vi "Paramater_analyser_main_file.vi"() -> ()   [LabVIEW 2021]
uses:
  <vilib>/Utility/file.llb/Write Delimited Spreadsheet (DBL).vi
panel:
  out "R-square":dbl format="%#_6e"
  out "Intercept":dbl format="%#_4e"
  out "Resistance (Ohm)":dbl format="%#_4p"
  in  "Estimated Length (mm)":dbl=12.0
  in  "Estimated Width (mm)":dbl=3.0
  out "Double - Voltage":dbl
  out "Double - Current":dbl
  out "First Cycle Reverse Sweep":cluster{"Y":dbl[], "Y":dbl[]}[](graph)
  out "First Cycle Forward Sweep":cluster{"Y":dbl[], "Y":dbl[]}[](graph)
  out "Single - Current":dbl
  out "Single - Voltage":dbl
  out "Recorded_Data":dbl[][][](array[numeric])
  out "WarmUp":dbl[][](array[numeric])
  out "Values Committed":bool
  in  "Press to start":bool
  in  "Set Swe_2_Mode":string(combo)="Single"
  in  "Set Swe_1_Mode":string(combo)="Double"
  in  "SMU1 Terminal":string(combo)="Source"
  in  "Sample Information":string="Synthetic_for_finishing program"
  in  "User":string="Richard"
  out "error out":errorcluster
  in  "VISA resource name":refnum<visa-resource-name>="PA"
  out "DorG_2":string
  out "DorG_1":string
  in  "VIntegration_2":dbl=100.0
  in  "VIntegration_1":dbl=100.0
  out "V_Cst_2 [V]":dbl
  out "V Cst_1 [V]":dbl
  out "V Cst_0 [V]":dbl
  out "V Step_2":dbl
  out "V Step_1":dbl
  out "V Step_0":dbl
  in  "Vvar_2_points":dbl=10.0
  in  "Vvar_1_points":dbl=10.0
  in  "Vvar_0_points":dbl=10.0
  in  "DorG_0":string(combo)="Gate"
  in  "Vvar_2_Stop":dbl=1.0
  in  "Vvar_1_Stop":dbl=1.0
  in  "Vvar_0_Stop":dbl
  in  "Vvar_2_start":dbl
  in  "Vvar_1_start":dbl
  in  "Vvar_0_start":dbl
  in  "# Cycles":dbl=1.0
  in  "Sweep Spacing_2":string(combo)="Linear"
  in  "Sweep Spacing_1":string(combo)="Linear"
  in  "Sweep Spacing_0":string(combo)="Linear"
  in  "VIntegration_0":dbl=100.0
  in  "Gate Current Compliance 2":dbl=1e-06
  in  "Gate Current Compliance 1":dbl=1e-06
  in  "Gate Current Compliance 0":dbl=1e-06
  in  "Drain Current Compliance 2":dbl=0.0001 format="%#_6p"
  in  "Drain Current Compliance 1":dbl=0.01 format="%#_6p"
  in  "Drain Current Compliance":dbl=1e-06
  in  "Sweep 2":bool
  in  "Sweep 0":bool
  in  "Vvar-2_delaytime":dbl
  in  "Vvar_1_delaytime":dbl
  in  "Vvar-0_delaytime":dbl
  in  "Vvar_2_holdtime":dbl
  in  "Vvar_1_holdtime":dbl
  in  "Vvar_0_holdtime":dbl
  out "VISA resource name out":refnum<visa-resource-name>
  in  "error in (no error)":errorcluster
  out "SMU3 Terminal":string
  out "SMU2 Terminal":string
  out "Sweep 2 Point Checker":string
  out "Sweep 2 Pot Check":string
  out "Sweep 1 Point Checker":string
  out "Sweep 1 Pot Check":string
  out "Gate Point number Checker":string
  out "Gate Potential_checker":string
  in  "V_const_2":dbl
  in  "V_const_1":dbl
  in  "V_const_0":dbl
  in  "Vstep2":dbl
  in  "Vstep1":dbl
  in  "Vstep0":dbl
  # "Meta Data"
  # "I(S)"
  # "I(G)"
  # "Voltage"
  # "T(G)"
  # "T(S)"
  # "T(D)"
  # "I(D)"
  # "Warmup is not yet fully implemented"
  # "V Stop"
  # "Sweep Mode"
  # "Delay Time"
  # "Drain/Gate"
  # "V Start"
  # "# Points"
  # "V Step"
  # "V Cst"
  # "Sweep Spacing"
  # "Drain Current Comp"
  # "Gate Current Comp"
  # "Hold Time"
  # "Integration"
  # "Single"
  # "V Stop"
  # "Sweep Mode"
  # "Delay Time"
  # "Drain/Gate"
  # "V Start"
  # "# Points"
  # "V Step"
  # "V Cst"
  # "Sweep Spacing"
  # "Drain Current Comp"
  # "Gate Current Comp"
  # "Hold Time"
  # "Integration"
  # "Operational_placeholders do not modify"
  # "Second_sweep is not yet implemented"
  # "V Stop"
  # "Sweep Mode"
  # "Delay Time"
  # "Drain/Gate"
  # "V Start"
  # "# Points"
  # "V Step"
  # "V Cst"
  # "Sweep Spacing"
  # "Drain Current Comp"
  # "Gate Current Comp"
  # "Hold Time"
  # "Integration"
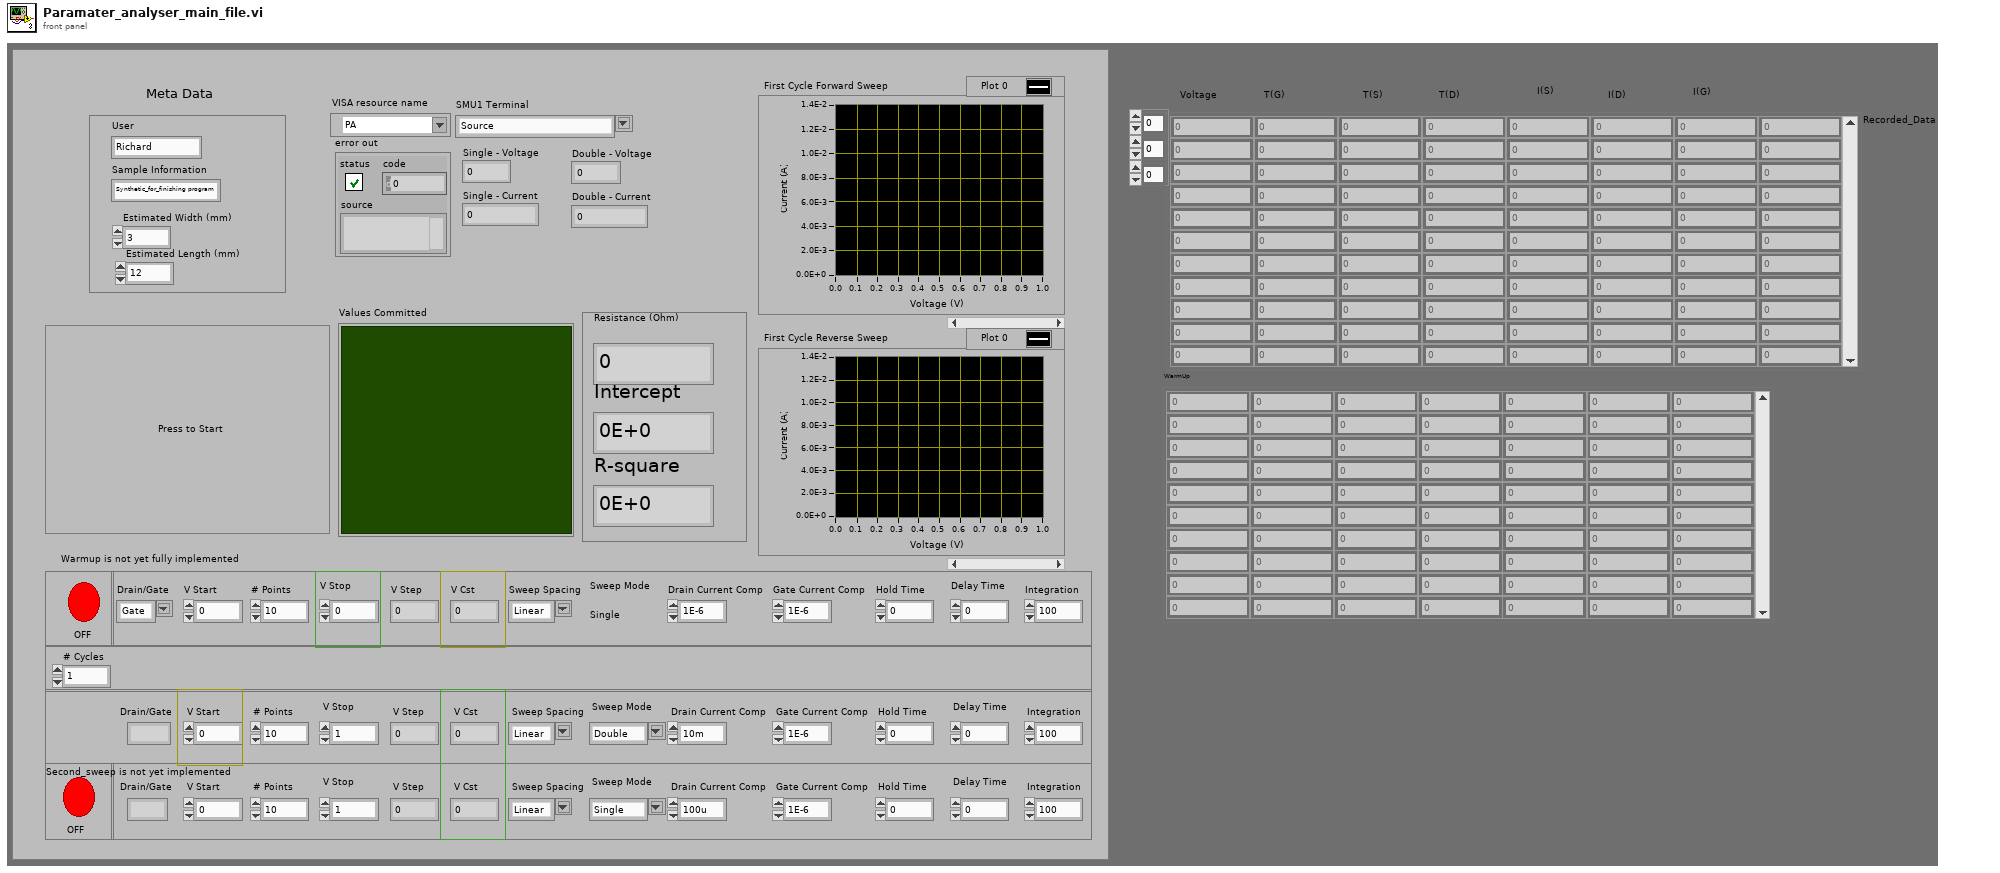
[diagram p1: front panel]
types:
  T1 = enum16{"open", "replace", "create", "open or create", "replace or create", "replace or create with confirmation"}
  T2 = cluster{"DorG_0":string, "Vvar_0_start":dbl, "Vstep0":dbl, "Vvar_0_Stop":dbl, "V_const_0":dbl, "Drain Current Compliance":dbl, "Gate Current Compliance 0":dbl, "Vvar_0_holdtime":dbl, "Vvar-0_delaytime":dbl, "Output Integration":dbl, string, "Sweep Spacing_0":string}
  T3 = cluster{string, "Vvar_1_start ":dbl, "Vstep1":dbl, "Vvar_1_Stop":dbl, "V_const_1":dbl, "Drain Current Compliance 1":dbl, "Gate Current Compliance 1":dbl, "Vvar_1_holdtime":dbl, "Vvar_1_delaytime":dbl, "Output Integration":dbl, "Set Swe_1_Mode":string, "Sweep Spacing_1":string}
  T4 = cluster{string, "Vvar_2_start":dbl, "Vstep2":dbl, "Vvar_2_Stop":dbl, "V_const_2":dbl, "Drain Current Compliance 2":dbl, "Gate Current Compliance 2":dbl, "Vvar_2_holdtime":dbl, "Vvar-2_delaytime":dbl, "Output Integration":dbl, "Set Swe_2_Mode":string, "Sweep Spacing_2":string}
  T5 = cluster{"DorG":string, "Vvar_start":dbl, "Vvar_step":dbl, "Vvar_Stop":dbl, "V_const ":dbl, "Drain Current Compliance":dbl, "Gate Current Compliance":dbl, "Vvar_holdtime":dbl, "Vvar_delaytime":dbl, "IntPts":dbl, "Set Swe_Mode":string, "Sweep Spacing":string}
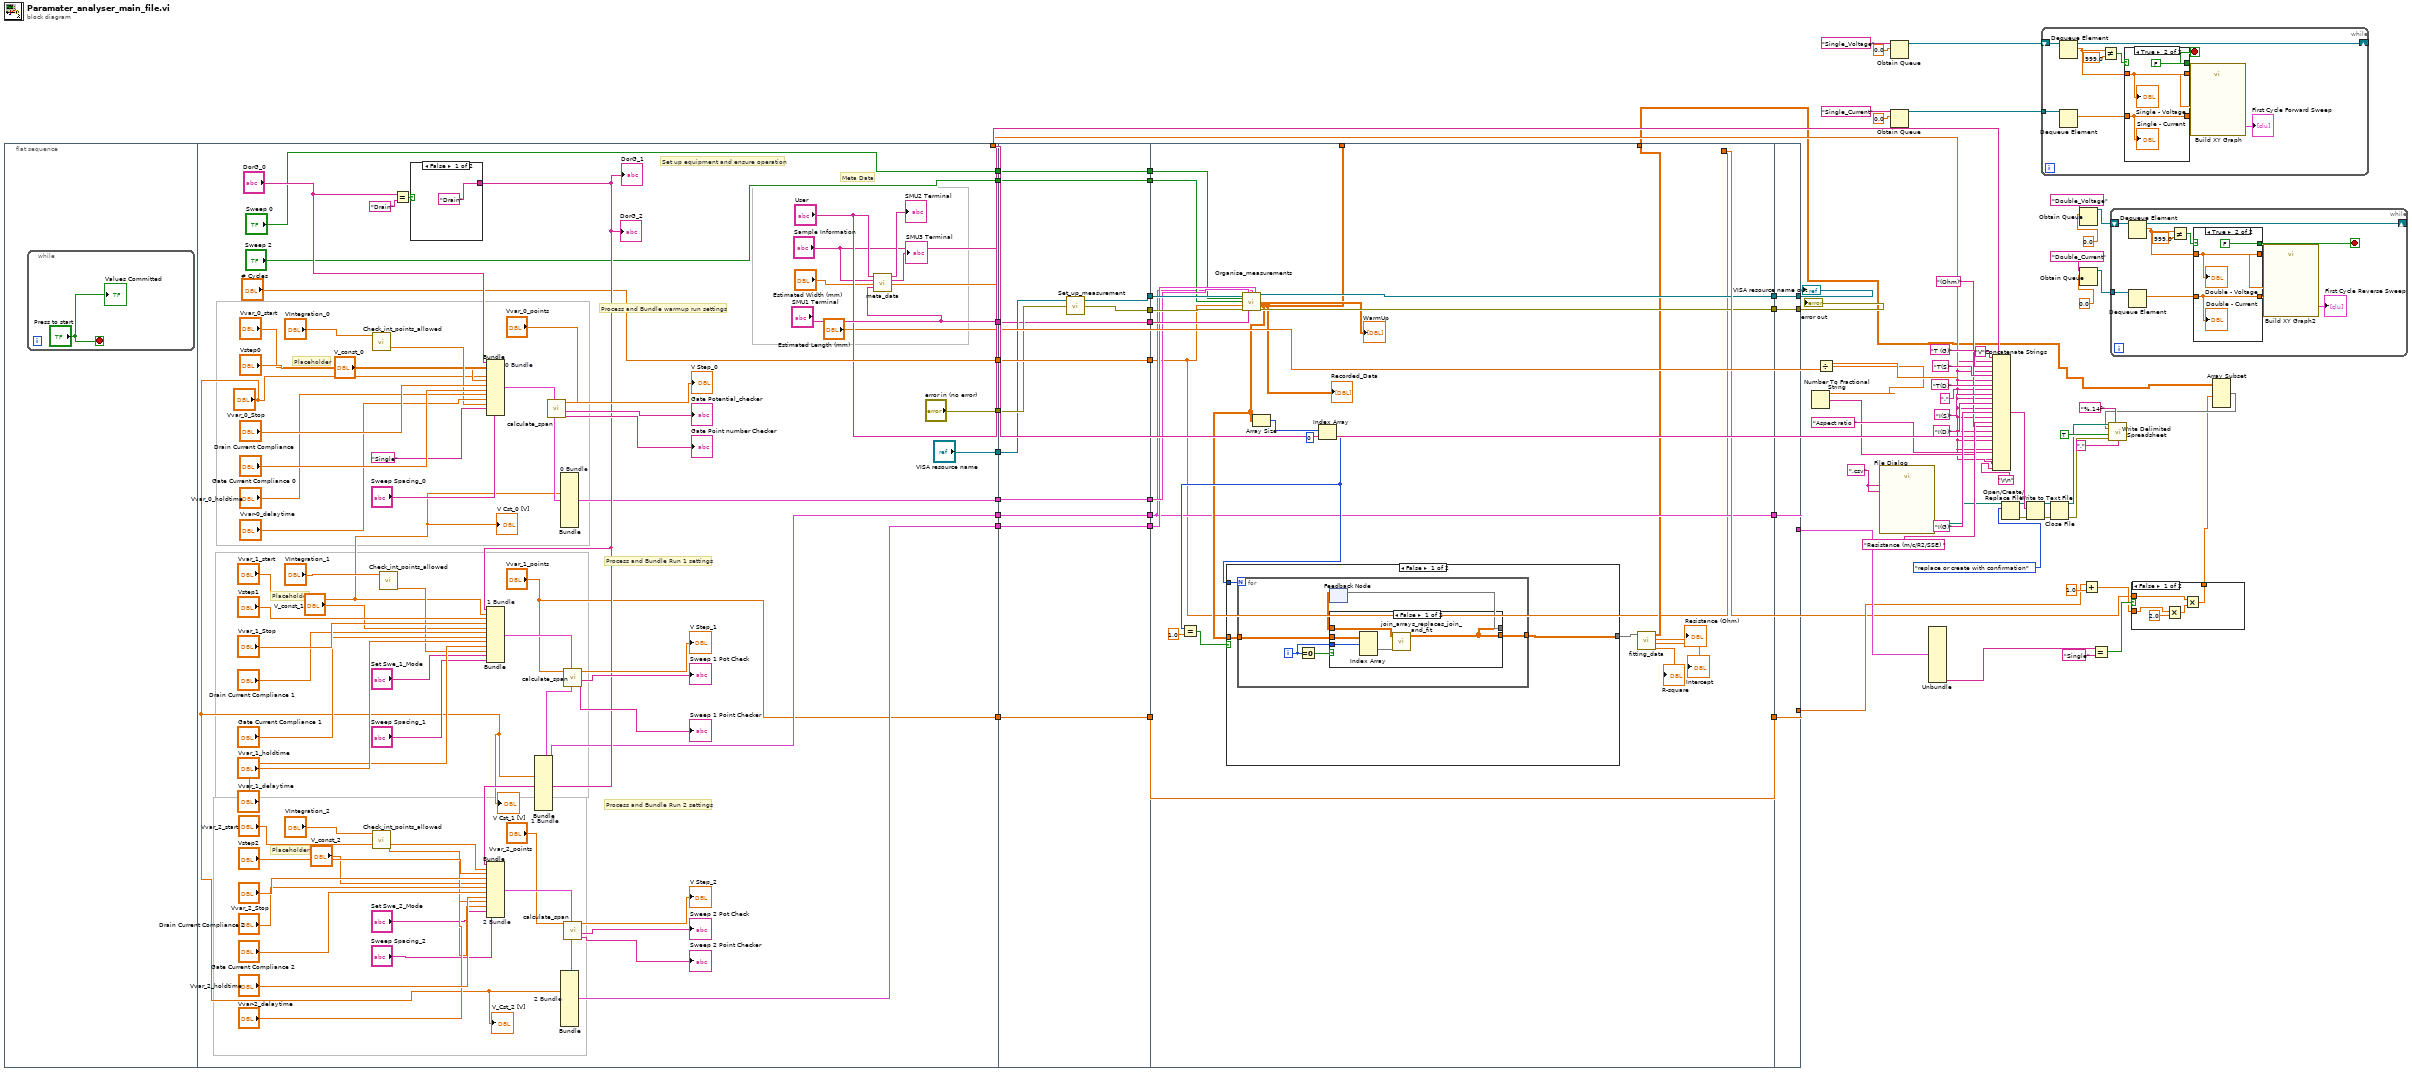
[diagram p0: block diagram]
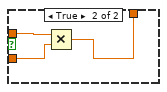
[diagram p2: hidden frame]
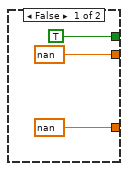
[diagram p3: hidden frame]
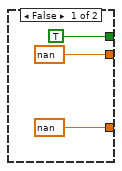
[diagram p4: hidden frame]
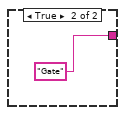
[diagram p5: hidden frame]
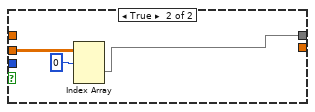
[diagram p6: hidden frame]
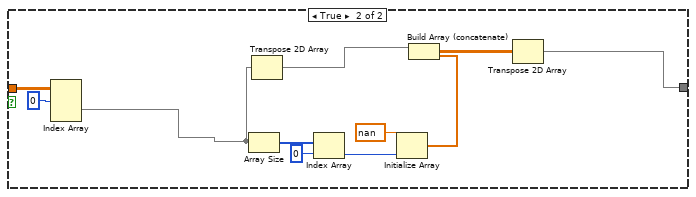
[diagram p7: hidden frame]
diagram:
  w2 = "," ("string")
  w40 = ".csv" ("pattern (all files)")
  n1 = flat-sequence {
    tunnel: ["# Cycles"] -> w78
    tunnel: ["error in (no error)"] -> w74
    tunnel: ["VISA resource name"] -> w73
    tunnel: ["SMU1 Terminal"] -> w72
    tunnel: [w92] -> w70
    tunnel: [w91] -> w68
    tunnel: [w90] -> w66
    tunnel: ["Sweep 2"] -> w64
    tunnel: ["Sweep 0"] -> w62
    tunnel: ["User"] -> w31
    tunnel: ["Sample Information"] -> w30
    tunnel: ["Estimated Width (mm)"] -> w22
    tunnel: ["Estimated Length (mm)"] -> w21
    tunnel: ["Vvar_1_points"] -> w9
    tunnel: w78 -> [w168]
    tunnel: [w168] -> w77
    tunnel: [w167] -> w76
    tunnel: [w166] -> w75
    tunnel: w74 -> [w165]
    tunnel: w73 -> [w164]
    tunnel: w72 -> [w163]
    tunnel: [w163] -> w71
    tunnel: w70 -> [w162]
    tunnel: [w162] -> w69
    tunnel: w68 -> [w161]
    tunnel: [w161] -> w67
    tunnel: w66 -> [w160]
    tunnel: [w160] -> w65
    tunnel: w64 -> [w159]
    tunnel: [w159] -> w63
    tunnel: w62 -> [w158]
    tunnel: [w158] -> w61
    tunnel: [w157] -> w10
    tunnel: w9 -> [w157]
    tunnel: w77 -> [w172]
    tunnel: w76 -> [w190]
    tunnel: w75 -> [w189]
    tunnel: w71 -> [w188]
    tunnel: w69 -> [w187]
    tunnel: w67 -> [w176]
    tunnel: w65 -> [w186]
    tunnel: w63 -> [w185]
    tunnel: w61 -> [w184]
    tunnel: [w192] -> w60
    tunnel: [w191] -> w59
    tunnel: [w173] -> w18
    tunnel: [w177] -> _
    tunnel: [w176] -> w16
    tunnel: w10 -> [w175]
    tunnel: [w175] -> w8
    tunnel: [w172] -> w1
    tunnel: [w223] -> w79
    tunnel: [w224] -> w80
    tunnel: w60 -> [w224]
    tunnel: w59 -> [w223]
    tunnel: w16 -> [w222]
    tunnel: [w222] -> w15
    tunnel: w8 -> [w221]
    tunnel: [w221] -> w6
    frame #0 {
      n2 = while {
        stop <- "Press to start" stop-if-true
        "Values Committed" <- "Press to start"
      }
    }
    frame #1 {
      # "Set up equipment and ensure operation"
      # "Meta Data"
      # "Process and Bundle warmup run settings"
      # "Process and Bundle Run 1 settings"
      # "Process and Bundle Run 2 settings"
      # "Placeholder"
      # "Placeholder"
      # "Placeholder"
      n3 = call "Check_int_points_allowed.vi"("Integration Points"="VIntegration_0") -> ("Output Integration"=w136:dbl)  [unwired: 9 in, 1 out]
      n4 = call "Check_int_points_allowed.vi"("Integration Points"="VIntegration_2") -> ("Output Integration"=w106:dbl)  [unwired: 9 in, 1 out]
      n5 = call "Check_int_points_allowed.vi"("Integration Points"="VIntegration_1") -> ("Output Integration"=w119:dbl)  [unwired: 9 in, 1 out]
      n6 = Equal?(x="DorG_0", y="Drain") -> (x = y?=w152:bool)
      n7 = case shown="False" w152 {
        tunnel: ["Drain" "Gate"] -> w116
        frame False {
        }
        frame True {
        }
      }
      "DorG_1" <- w116
      "DorG_2" <- w116
      n8 = Bundle "0 Bundle"("DorG_0"="DorG_0", "Vvar_0_start"="Vvar_0_start", "Vstep0"="Vstep0", "Vvar_0_Stop"="Vvar_0_Stop", "V_const_0"="V_const_0", "Drain Current Compliance"="Drain Current Compliance", "Gate Current Compliance 0"="Gate Current Compliance 0", "Vvar_0_holdtime"="Vvar_0_holdtime", "Vvar-0_delaytime"="Vvar-0_delaytime", "Output Integration"=w136, "Single", "Sweep Spacing_0"="Sweep Spacing_0") -> (w130:T2)  [unwired: 1 in]
      n9 = Bundle "1 Bundle"(w116, "Vvar_1_start"="Vvar_1_start", "Vstep1"="Vstep1", "Vvar_1_Stop"="Vvar_1_Stop", "V_const_1"="V_const_1", "Drain Current Compliance 1"="Drain Current Compliance 1", "Gate Current Compliance 1"="Gate Current Compliance 1", "Vvar_1_holdtime"="Vvar_1_holdtime", "Vvar_1_delaytime"="Vvar_1_delaytime", "Output Integration"=w119, "Set Swe_1_Mode"="Set Swe_1_Mode", "Sweep Spacing_1"="Sweep Spacing_1") -> (w126:T3)  [unwired: 1 in]
      n10 = Bundle "2 Bundle"(w116, "Vvar_2_start"="Vvar_2_start", "Vstep2"="Vstep2", "Vvar_2_Stop"="Vvar_2_Stop", "V_const_2"="V_const_2", "Drain Current Compliance 2"="Drain Current Compliance 2", "Gate Current Compliance 2"="Gate Current Compliance 2", "Vvar_2_holdtime"="Vvar_2_holdtime", "Vvar-2_delaytime"="Vvar-2_delaytime", "Output Integration"=w106, "Set Swe_2_Mode"="Set Swe_2_Mode", "Sweep Spacing_2"="Sweep Spacing_2") -> (w114:T4)  [unwired: 1 in]
      n11 = call "calculate_span.vi"("Sweep in"=w130, "V_points"="Vvar_0_points") -> ("Gate Point number Checker"=→"Gate Point number Checker":string, "Gate Potential_checker"=→"Gate Potential_checker":string, "V Step"=→"V Step_0":dbl, "Sweep out"=w129:T5)  [unwired: 6 in]
      n12 = Bundle "0 Bundle"(cluster=w129, "V_const"="Vvar_1_start") -> (w92:T5)  [unwired: 11 in]
      n13 = call "calculate_span.vi"("Sweep in"=w126, "V_points"="Vvar_1_points") -> ("Gate Point number Checker"=→"Sweep 1 Point Checker":string, "Gate Potential_checker"=→"Sweep 1 Pot Check":string, "V Step"=→"V Step_1":dbl, "Sweep out"=w125:T5)  [unwired: 6 in]
      n14 = Bundle "1 Bundle"(cluster=w125, "V_const"="Vvar_0_Stop") -> (w91:T5)  [unwired: 11 in]
      n15 = call "calculate_span.vi"("Sweep in"=w114, "V_points"="Vvar_2_points") -> ("Gate Point number Checker"=→"Sweep 2 Point Checker":string, "Gate Potential_checker"=→"Sweep 2 Pot Check":string, "V Step"=→"V Step_2":dbl, "Sweep out"=w113:T5)  [unwired: 6 in]
      n16 = Bundle "2 Bundle"(cluster=w113, "V_const"="Vvar_0_Stop") -> (w90:T5)  [unwired: 11 in]
      n17 = call "meta_data.vi"("User"="User", "Sample Information"="Sample Information", "SMU1 Terminal"="SMU1 Terminal") -> ("SMU2 Terminal"=→"SMU2 Terminal":string, "SMU3 Terminal"=→"SMU3 Terminal":string)  [unwired: 11 in]
      "V Cst_0 [V]" <- "Vvar_1_start"
      "V Cst_1 [V]" <- "Vvar_0_Stop"
      "V_Cst_2 [V]" <- "Vvar_0_Stop"
    }
    frame #2 {
      n18 = call "Set_up_measurement.vi"("error in (no error)"=w165, "VISA resource name"=w164) -> ("error out"=w167:errorcluster, "VISA resource name out"=w166:refnum<visa-resource-name>)  [unwired: 2 in]
    }
    frame #3 {
      n19 = call "Organise_measurements.vi"("VISA resource name"=w189, 1:"Sweep 0"=w187, "Sweep 1_replac"=w176, "Sweep 2_replac 2"=w186, 5:"Sweep 0"=w184, "Sweep 2"=w185, "# Cycles"=w172, "error in (no error)"=w190, "SMU1 Terminal"=w188) -> ("VISA resource name out"=w192:refnum<visa-resource-name>, "WarmUp"=→"WarmUp":dbl[][], "Recorded_Data"=w177:dbl[][][], "error out"=w191:errorcluster)  [unwired: 3 in]
      "Recorded_Data" <- w177
      n20 = Array Size(array=w177) -> (size(s)=w182:i32[])
      n21 = Index Array(array=w182, index=0) -> (element=w178:i32)
      n22 = Equal?(x=w178, y=1.0) -> (x = y?=w179:bool)
      n23 = case shown="False" w179 {
        tunnel: w177 -> [w194 w219]
        tunnel: [w193 w211] -> w174
        tunnel: w178 -> [w195 _]
        frame False {
          n24 = for {
            N: w195 -> [_]
            tunnel: w194 -> [w200]
            tunnel: [w196] -> w193
            i -> [w197]
            n25 = Equal To 0?(x=w197) -> (x = 0?=w201:bool)
            n26 = feedback #1() -> (w198:dbl[][])  [unwired: 1 in]
            n27 = case shown="False" w201 {
              tunnel: w200 -> [w205 w209]
              tunnel: [w202 w207] -> w199
              tunnel: w198 -> [w206 _]
              tunnel: w197 -> [w204 _]
              tunnel: [w202 _] -> w196
              frame False {
                n28 = Index Array(array=w205, index (dim 0)=w204) -> (element=w203:dbl[][])  [unwired: 2 in]
                n29 = call "join_arrays_replaces_join_and_fit.vi"("Array to be added"=w203, "Old Array"=w206) -> ("Output array"=w202:dbl[][])  [unwired: 9 in]
              }
              frame True {
                n30 = Index Array(array=w209, index (dim 0)=0 ("index (page)")) -> (element=w207:dbl[][])  [unwired: 2 in]
              }
            }
            n31 = feedback-in #1(w199) -> ()
          }
        }
        frame True {
          n32 = Index Array(array=w219, index (dim 0)=0 ("index (page)")) -> (element=w210:dbl[][])  [unwired: 2 in]
          n33 = Array Size(array=w210) -> (size(s)=w218:i32[])
          n34 = Transpose 2D Array(2D array=w210) -> (transposed array=w214:dbl[][])
          n35 = Index Array(array=w218, index=0) -> (element=w215:i32)
          n36 = Initialize Array(nan ("element"), w215) -> (w213:dbl[])
          n37 = Build Array (concatenate)(w214, w213) -> (w212:dbl[][])
          n38 = Transpose 2D Array(2D array=w212) -> (transposed array=w211:dbl[][])
        }
      }
      n39 = call "fitting_data.vi"("Recorded_Data 2"=w174) -> ("R-square"=→"R-square":dbl, "intercept"=→"Intercept":dbl, "slope"=→"Resistance (Ohm)":dbl, "Recorded_Data 3"=w173:dbl[][])  [unwired: 3 in]
    }
    frame #4 {
    }
  }
  n40 = Divide(x=w22, y=w21) -> (x/y=w19:dbl)
  n41 = Number To Fractional String(number=w19) -> (F-format string=w3:string)  [unwired: 3 in]
  n42 = call "File Dialog"("pattern (all files)"=w40, "pattern label"=w40) -> ("selected path"=w39:path)  [unwired: 10 in, 3 out]
  n43 = Obtain Queue(name (unnamed)="Single_Voltage", element data type=0.0) -> (queue out=w56:refnum<queue>)  [unwired: 3 in, 2 out]
  n44 = Obtain Queue(name (unnamed)="Single_Current", element data type=0.0) -> (queue out=w53:refnum<queue>)  [unwired: 3 in, 2 out]
  n45 = Unbundle(w15) -> ("Sweep Spacing"=w14:string)  [unwired: 11 out]
  n46 = Concatenate Strings("V" ("string"), w2, "T (G)" ("string"), w2, "T(S)" ("string"), w2, "T(D)" ("string"), w2, "I(S)" ("string"), w2, "I(D)" ("string"), w2, "I(G)" ("string"), w2, "Resistance (m/c/R2/SSE) " ("string"), "(Ohm)" ("string"), w2, w31, w2, w30, w2, "Aspect ratio " ("string"), w2, w3, "\r\n") -> (w41:string)
  n47 = Open/Create/Replace File(file path (use dialog)=w39, operation (0:open)=T1."replace or create with confirmation") -> (refnum out=w34:refnum<file>, error out=w35:errorcluster)  [unwired: 4 in, 1 out]
  n48 = Write to Text File(file (use dialog)=w34, text=w41, error in=w35) -> (refnum out=w37:refnum<file>, error out=w36:errorcluster)  [unwired: 1 in, 1 out]
  n49 = while {
    shift-right: [w234] -> _
    shift-left: w56 -> [w235]
    tunnel: w53 -> [w229]
    stop <- w233 stop-if-true
    n50 = Dequeue Element(queue=w235) -> (queue out=w234:refnum<queue>, element=w231:dbl)  [unwired: 2 in, 2 out]
    n51 = Dequeue Element(queue=w229) -> (element=w228:dbl)  [unwired: 2 in, 3 out]
    n52 = Not Equal?(x=w231, y=999.0) -> (x != y?=w230:bool)
    n53 = case shown="True" w230 {
      tunnel: w231 -> [_ w240]
      tunnel: [TRUE FALSE] -> w233
      tunnel: [nan w240] -> w226
      tunnel: w228 -> [_ w239]
      tunnel: [nan w239] -> w225
      frame False {
      }
      frame True {
        "Single - Voltage" <- w240
        "Single - Current" <- w239
      }
    }
    n54 = call "Build XY Graph"("Y Input"=w225, "X Input"=w226) -> ("XY Graph"=→"First Cycle Forward Sweep":cluster{"X":dbl[], "Y":dbl[]}[])  [unwired: 8 in, 1 out]
  }
  n55 = Close File(refnum=w37, error in=w36) -> (path=w49:path, error out=w50:errorcluster)
  n56 = Obtain Queue(name (unnamed)="Double_Voltage", element data type=0.0) -> (queue out=w27:refnum<queue>)  [unwired: 3 in, 2 out]
  n57 = Obtain Queue(name (unnamed)="Double_Current", element data type=0.0) -> (queue out=w24:refnum<queue>)  [unwired: 3 in, 2 out]
  n58 = Add(x=w6, y=1.0) -> (x+y=w5:dbl)
  n59 = Equal?(x=w14, y="Single") -> (x = y?=w11:bool)
  n60 = while {
    shift-right: [w251] -> _
    shift-left: w27 -> [w252]
    tunnel: w24 -> [w246]
    stop <- w250 stop-if-true
    n61 = Dequeue Element(queue=w252) -> (queue out=w251:refnum<queue>, element=w248:dbl)  [unwired: 2 in, 2 out]
    n62 = Dequeue Element(queue=w246) -> (element=w245:dbl)  [unwired: 2 in, 3 out]
    n63 = Not Equal?(x=w248, y=999.0) -> (x != y?=w247:bool)
    n64 = case shown="True" w247 {
      tunnel: w248 -> [_ w257]
      tunnel: [TRUE FALSE] -> w250
      tunnel: [nan w257] -> w243
      tunnel: w245 -> [_ w256]
      tunnel: [nan w256] -> w242
      frame False {
      }
      frame True {
        "Double - Voltage" <- w257
        "Double - Current" <- w256
      }
    }
    n65 = call "Build XY Graph2"("Y Input"=w242, "X Input"=w243) -> ("XY Graph"=→"First Cycle Reverse Sweep":cluster{"X":dbl[], "Y":dbl[]}[])  [unwired: 8 in, 1 out]
  }
  n66 = case shown="False" w11 {
    tunnel: [w261 w266] -> w12
    tunnel: w5 -> [w262 w265]
    tunnel: w1 -> [w259 w264]
    frame False {
      n67 = Multiply(x=w262, y=2.0) -> (x*y=w260:dbl)
      n68 = Multiply(x=w259, y=w260) -> (x*y=w261:dbl)
    }
    frame True {
      n69 = Multiply(x=w264, y=w265) -> (x*y=w266:dbl)
    }
  }
  n70 = Array Subset(array=w18, length (row)=w12) -> (w17:dbl[][])  [unwired: 3 in]
  n71 = call-poly <vilib>:"Write Delimited Spreadsheet.vi"("file path (dialog if empty)"=w49, "format (%.3f)"="%.14f", "2D data"=w17, "append to file? (new file:F)"=TRUE, "error in (no error)"=w50, "delimiter (\\t)"="," ("delimiter (\\t)")) -> ()  [unwired: 8 in, 2 out]
  "error out" <- w79
  "VISA resource name out" <- w80
